vi "Set ObjectType.vi"(8 "error in":errorcluster, 10 "ObjectType":refnum<class "Value.lvclass">, 11 "Object Type in":refnum<class "Object Type Base.lvclass">) -> (0 "error out":errorcluster, 3 "Object Type out":refnum<class "Object Type Base.lvclass">)   [LabVIEW 2019, in "Electronic Datasheet.lvlib" / "Object Type Base.lvclass"]
uses:
  Object Type Base.lvclass
  Value/Value.lvclass
  Object Type Base.lvclass/Object Type Base.ctl
  Object Type.ctl
  Electronic Datasheet.lvlib
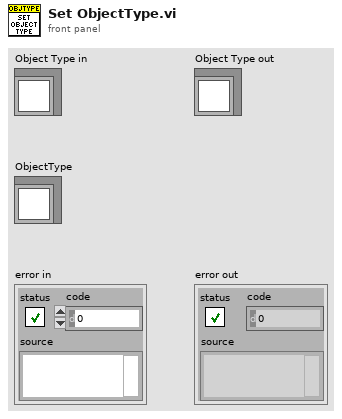
[diagram p1: front panel]
types:
  T1 = typedef "Electronic Datasheet.lvlib/Object Type.ctl" = u8
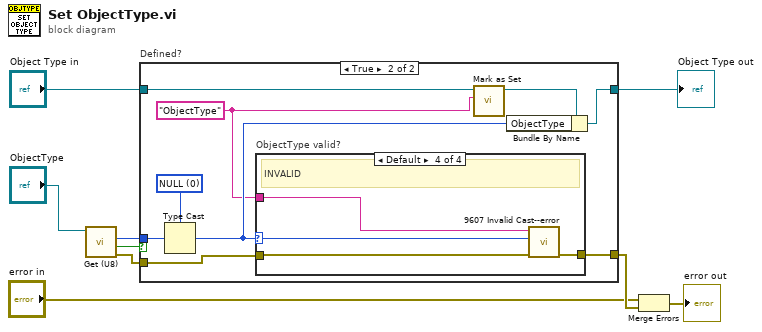
[diagram p0: block diagram]
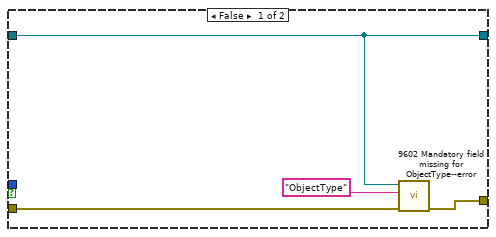
[diagram p2: hidden frame]
diagram:
  n1 = call "Get (U8).vi"("Value in"="ObjectType") -> ("error out"=w4:errorcluster, "Defined?"=w6:bool, "Value"=w5:u8)  [unwired: 7 in, 1 out]
  n2 = case "Defined?" shown="True" w6 {
    tunnel: [w10 w22] -> w9
    tunnel: "Object Type in" -> [w10 w21]
    tunnel: w5 -> [_ w18]
    tunnel: w4 -> [w13 w15]
    tunnel: [w12 w19] -> w3
    frame False {
      n3 = call "9602 Mandatory field missing for ObjectType--error.vi"("error in"=w13, "Field Name"="ObjectType" ("error message (\"\")"), "Object Type Base"=w10) -> ("error out"=w12:errorcluster)  [unwired: 8 in]
    }
    frame True {
      w17 = T1 0 items=["NULL"=0, "DOMAIN"=2, "DEFTYPE"=5, "DEFSTRUCT"=6, "VAR"=7, "ARRAY"=8, "RECORD"=9] ("ObjectType")
      w14 = "ObjectType" ("Field name")
      n4 = Type Cast(type=w17, x=w18) -> (*(type *) &x=w16:T1)
      n5 = case "ObjectType valid?" shown="Default" w16 {
        selector: w16 -> [_ _ _ w26]
        tunnel: w15 -> [w23 w24 w25 w28]
        tunnel: [w23 w24 w25 w29] -> w19
        tunnel: w14 -> [_ _ _ w27]
        frame 0 {
          # "NULL"
        }
        frame 2 {
          # "DOMAIN"
        }
        frame 5..9 {
          # "VALIDS"
        }
        frame Default {
          # "INVALID"
          n6 = call "9607 Invalid Cast--error.vi"("error in"=w28, "Value"=w26, "Type"=w27) -> ("error out"=w29:errorcluster)  [unwired: 8 in]
        }
      }
      n7 = call "Mark as Set.vi"("Field name"=w14, "Object Type in"=w21) -> ("Object Type out"=w20:refnum<class "Object Type Base.lvclass">)  [unwired: 9 in]
      n8 = Bundle By Name(cluster=w20, "ObjectType"=w16) -> (w22:refnum<class "Object Type Base.lvclass">)
    }
  }
  "Object Type out" <- w9
  n9 = Merge Errors("error in", w3) -> (→"error out":errorcluster)
